vi "Linear search in case of collisions.vi"(10 "Constant Name":string, 11 "Array":T1[](array[typedef])) -> (0 "index":i32, 2 "Did it find it":bool, 3 "Constants":T1)   [LabVIEW 2013]
uses:
  Constants typedef V2.ctl
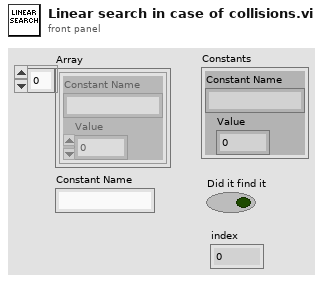
[diagram p1: front panel]
types:
  T1 = typedef "Constants typedef V2.ctl" = cluster{"Constant Name":string, "Value":dbl}
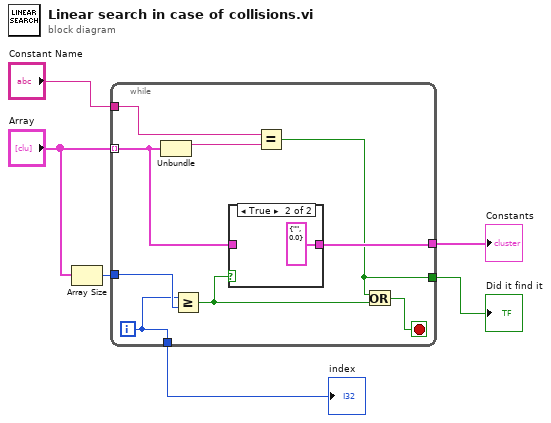
[diagram p0: block diagram]
diagram:
  n1 = Array Size(array="Array") -> (size(s)=w5:i32)
  n2 = while {
    tunnel: "Array" -> [w13] mode=indexing
    tunnel: "Constant Name" -> [w14]
    tunnel: [w10] -> w3
    tunnel: w5 -> [w12]
    tunnel: [w8] -> w6
    tunnel: [w7] -> w1
    i -> [w7]
    stop <- w11 stop-if-true
    n3 = Unbundle(w13) -> ("Constant Name"=w15:string)  [unwired: 1 out]
    n4 = Greater Or Equal?(x=w7, y=w12) -> (x >= y?=w9:bool)
    n5 = case shown="True" w9 {
      tunnel: w13 -> [w16 _]
      tunnel: [w16 T1 {"Constant Name"="", "Value"=0.0} ("Constants")] -> w10
      frame False {
      }
      frame True {
      }
    }
    n6 = Equal?(x=w14, y=w15) -> (x = y?=w8:bool)
    n7 = Or(x=w8, y=w9) -> (x .or. y?=w11:bool)
  }
  "Did it find it" <- w6
  "Constants" <- w3
  "index" <- w1
